vi "u8Array.vi"(3 "Array Length":i32=-1, 4 "Array":u8[](array[numeric]), 5 "msg in":string) -> (2 "msg out":string)   [LabVIEW 2015]
panel:
  # "Array type is according to the ROS message definition.\n\nIf the array is declared \n               primitive[] name\nThe array is variable length\n\n\nIf the array is declared              \n               primitive[*] name\nthe array is fixed length"
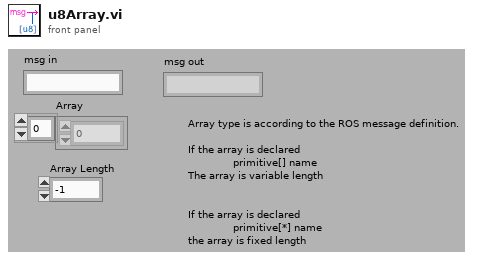
[diagram p1: front panel]
types:
  T1 = enum16{"big-endian, network order", "native, host order", "little-endian"}
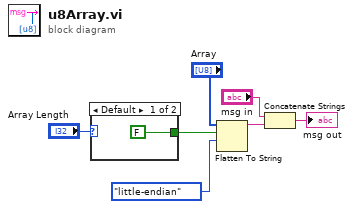
[diagram p0: block diagram]
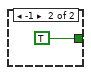
[diagram p2: hidden frame]
diagram:
  n1 = case shown="Default" "Array Length" {
    tunnel: [FALSE TRUE] -> w1
    frame Default {
    }
    frame -1 {
    }
  }
  n2 = Flatten To String(anything="Array", prepend array or string size? (T)=w1, byte order (0:big-endian, network order)=T1."little-endian") -> (data string=w6:string)  [unwired: 1 in, 2 out]
  n3 = Concatenate Strings("msg in", w6) -> (→"msg out":string)
